vi "Digital Write.vi"(8 "Error In":errorcluster, 9 "Values":bool[](array[boolean]), 10 "Channels":u8[](array[numeric]), 11 "LINX Device Config":T1) -> (0 "Error Out":errorcluster, 3 "LINX Device Config":T1)   [LabVIEW 2011, in "LMH-LINX.lvlib" / "Device.lvlib"]
doc: "Set the value of one or more digital output pin."
uses:
  Device.lvlib
  Type Defs/LINX Device Config.ctl
  Type Defs/Interface.ctl
  Type Defs/TCP Config.ctl
  Type Defs/Channels.ctl
  Type Defs/Error Type.ctl
  LMH-LINX.lvlib
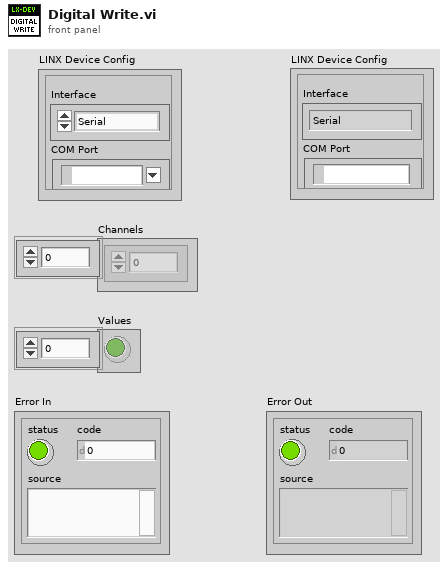
[diagram p1: front panel]
types:
  T1 = typedef "LMH-LINX.lvlib/Device.lvlib/LINX Device Config.ctl" = cluster{"Interface":T2, "COM Port":refnum<visa-resource-name>, "TCP Configuration":T3, "Device Family":u8, "Device ID":u8, "Device Name":string, "TCP Ref":refnum<k5>, "Channels":T4}
  T2 = typedef "LMH-LINX.lvlib/Interface.ctl" = enum16{"Serial", "TCP"}
  T3 = typedef "LMH-LINX.lvlib/Device.lvlib/TCP Config.ctl" = cluster{"IP Address":string, "Port":u16}
  T4 = typedef "LMH-LINX.lvlib/Channels.ctl" = cluster{"DI":u8[], "DO":u8[], "AI":u8[], "AO":u8[], "PWM":u8[], "QE":u8[], "UART":u8[], "I2C 2":u8[], "SPI":u8[], "CAN":u8[], "Servo":u8[], "AI Ref (V)":dbl, "AO Ref (V)":dbl, "AO Resolution (Bits)":u8}
  T5 = typedef "LMH-LINX.lvlib/Error Type.ctl" = enum16{"Unknown", "Timeout", "Corrupt Return Packet", "Unable To Connect", "Command Not Supported", "Channel DNE", "Invalid COM Config", "Firmware Version Mismatch", "myRIO Support", "CMD Specific Error"}
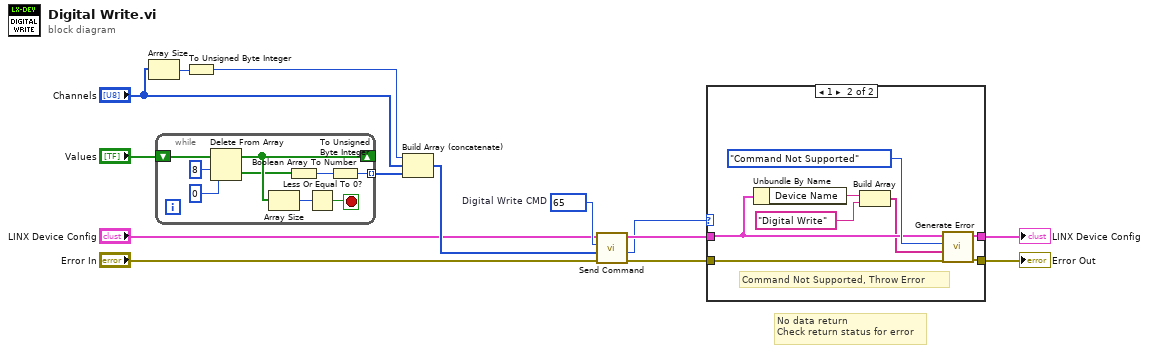
[diagram p0: block diagram]
diagram:
  w13 = u16 65  # Digital Write CMD
  # "No data return\nCheck return status for error"
  n1 = Array Size(array="Channels") -> (size(s)=w12:i32)
  n2 = while {
    shift-right: [w20] -> _
    shift-left: "Values" -> [w23]
    tunnel: [w15] -> w9 mode=indexing
    stop <- w18 stop-if-true
    n3 = Delete From Array(array=w23, length=8 ("index"), index=0 ("length")) -> (deleted portion=w17:bool[], array with subset deleted=w20:bool[])
    n4 = Array Size(array=w20) -> (size(s)=w19:i32)
    n5 = Boolean Array To Number(Boolean array=w17) -> (number=w16:u32)
    n6 = Less Or Equal To 0?(x=w19) -> (x <= 0?=w18:bool)
    n7 = To Unsigned Byte Integer(number=w16) -> (unsigned 8bit integer=w15:u8)
  }
  n8 = To Unsigned Byte Integer(number=w12) -> (unsigned 8bit integer=w11:u8)
  n9 = Build Array (concatenate)(w11, "Channels", w9) -> (w10:u8[])
  n10 = call "Send Command.vi"("Error In"="Error In", "ARGS"=w10, "CMD"=w13, "LINX Device Config"="LINX Device Config") -> ("Error Out"=w6:errorcluster, "Status"=w1:u8, "LINX Device Config"=w4:T1)  [unwired: 4 in, 1 out]
  n11 = case shown="1" w1 {
    tunnel: [w25 w31] -> w8
    tunnel: w4 -> [w25 w27]
    tunnel: [w24 w32] -> w7
    tunnel: w6 -> [w24 w33]
    frame 0, Default {
      # "Status OK"
    }
    frame 1 {
      # "Command Not Supported, Throw Error"
      n12 = Unbundle By Name(w27) -> ("Device Name"=w29:string)
      n13 = Build Array(w29, "Digital Write") -> (w26:string[])
      n14 = call "Generate Error.vi"("Error In"=w33, "Arguments"=w26, "Error Type"=Error_Type."Command Not Supported", "LINX Device Config"=w27) -> ("Error Out"=w32:errorcluster, "LINX Device Config"=w31:T1)  [unwired: 6 in]
    }
  }
  "Error Out" <- w7
  "LINX Device Config" <- w8
